vi "Automatic_light_attempt.vi"() -> ()   [LabVIEW 2019]
uses:
  <vilib>/MakerHub/LINX/Public/Peripherals/Analog/Analog Read 1 Chan.vi
  <vilib>/MakerHub/LINX/Public/Peripherals/Digital/Digital Write 1 Chan.vi
  <vilib>/MakerHub/LINX/Public/Peripherals/Analog/Analog Read N Chans.vi
  <vilib>/MakerHub/LINX/Public/Peripherals/Digital/Digital Write N Chans.vi
  <vilib>/MakerHub/LINX/Private/Local IO/LinxAnalogRead.vi
  <vilib>/MakerHub/LINX/Public/Utilities/Check Channel.vi
  <vilib>/MakerHub/LINX/Private/Local IO/LinxDigitalWrite.vi
  <vilib>/MakerHub/LINX/Public/Utilities/Open Serial.vi
  <vilib>/MakerHub/LINX/Private/Utilties/Generate Error.vi
  <vilib>/MakerHub/LINX/LMH-LINX.lvlib
panel:
  out "x < y?":bool
  out "Analog Output":dbl
  in  "stop":bool
  in  "Analog Channel":u8
  in  "Error In":errorcluster
  in  "Serial Port":refnum<visa-resource-name>="N/A"
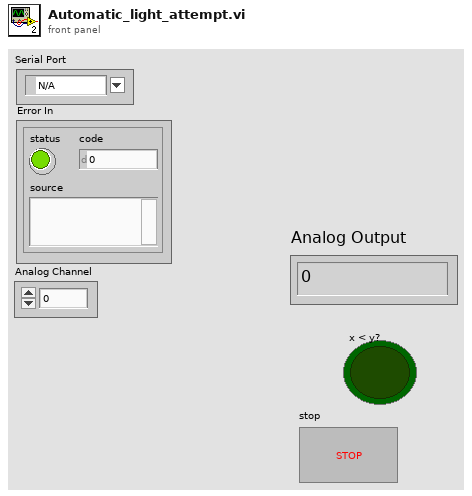
[diagram p1: front panel]
types:
  T1 = typedef "LMH-LINX.lvlib/LINX Ref.ctl" = cluster{"IO":T2, "Interface":T3, "LINX Device Config":T4}
  T2 = typedef "LMH-LINX.lvlib/Platform.ctl" = enum16{"Remote", "Local"}
  T3 = typedef "LMH-LINX.lvlib/Interface.ctl" = enum16{"Serial", "TCP"}
  T4 = typedef "LMH-LINX.lvlib/Device.lvlib/LINX Device Config.ctl" = cluster{"Interface":T3, "COM Port":refnum<visa-resource-name>, "TCP Configuration":T5, "Device Family":u8, "Device ID":u8, "Device Name":string, "TCP Ref":refnum<k5>, "Channels":T6}
  T5 = typedef "LMH-LINX.lvlib/Device.lvlib/TCP Config.ctl" = cluster{"IP Address":string, "Port":u16}
  T6 = typedef "LMH-LINX.lvlib/Channels.ctl" = cluster{"DI":u8[], "DO":u8[], "AI":u8[], "AO":u8[], "PWM":u8[], "QE":u8[], "UART":u8[], "I2C 2":u8[], "SPI":u8[], "CAN":u8[], "Servo":u8[], "AI Ref (V)":dbl, "AI Resolution (Bits)":u8, "AO Ref (V)":dbl, "AO Resolution (Bits)":u8}
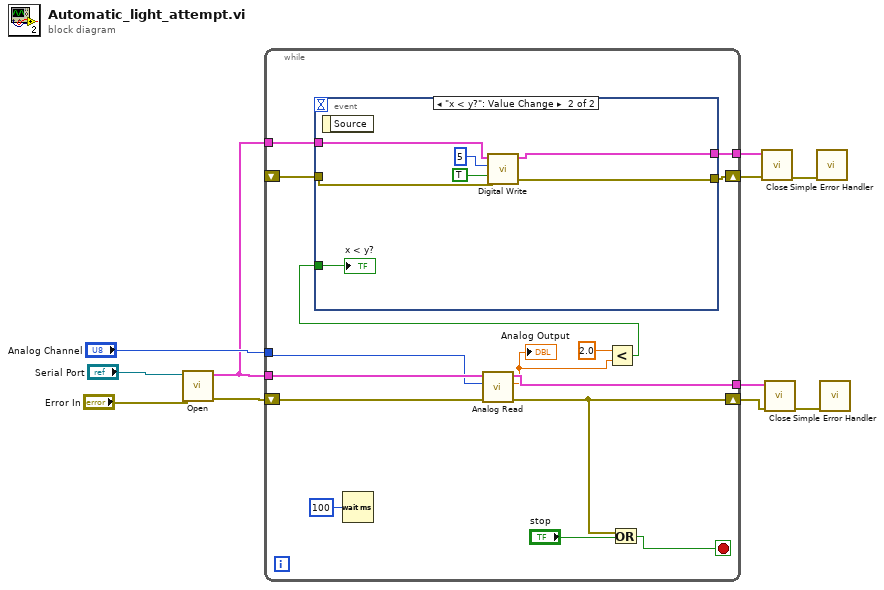
[diagram p0: block diagram]
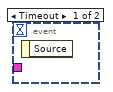
[diagram p2: hidden frame]
diagram:
  n1 = call-poly <vilib>:"Open.vi"("Error In"="Error In", "Serial Port"="Serial Port") -> ("Error Out"=w10:errorcluster, "LINX Resource"=w4:T1)  [unwired: 7 in, 1 out]
  n2 = while {
    tunnel: w4 -> [w26]
    tunnel: [w25] -> w11
    tunnel: "Analog Channel" -> [w23]
    shift-right: [w20] -> w9
    shift-left: w10 -> [w24]
    shift-right: [w15] -> w2
    shift-left: _ -> [w14]
    tunnel: w4 -> [w13]
    tunnel: [w12] -> w1
    stop <- w22 stop-if-true
    n3 = Wait (ms)(milliseconds to wait=u32 100) -> ()  [unwired: 1 out]
    n4 = call-poly <vilib>:"Analog Read.vi"("Error In"=w24, "Analog Channel"=w23, "LINX Resource"=w26) -> ("Error Out"=w20:errorcluster, "Voltage"=w18:dbl, "LINX Resource"=w25:T1)  [unwired: 5 in, 1 out]
    "Analog Output" <- w18
    n5 = Less?(x=2.0, y=w18) -> (x < y?=w16:bool)
    n6 = event shown="[1] \"x < y?\": Value Change" {
      selector: _ -> [_ _]
      dyn-events: _ -> [_ _]
      timeout: _ -> [_ _]
      tunnel: w16 -> [_ w33]
      tunnel: w14 -> [_ w32]
      tunnel: [_ w31] -> w15
      tunnel: w13 -> [_ w28]
      tunnel: [_ w27] -> w12
      event Timeout {
        n7 = event-data() -> ()  [unwired: 1 in, 1 out]
      }
      event "x < y?": Value Change {
        n8 = event-data() -> ()  [unwired: 1 in, 1 out]
        n9 = call-poly <vilib>:"Digital Write.vi"("Error In"=w32, "Output Value"=TRUE, "DO Channel"=u8 5, "LINX Resource"=w28) -> ("Error Out"=w31:errorcluster, "LINX Resource"=w27:T1)  [unwired: 6 in]
        "x < y?" <- w33
      }
    }
    n10 = Or(x=w20, y="stop") -> (x .or. y?=w22:bool)
  }
  n11 = call <vilib>:"Close.vi"("Error In"=w2, "LINX Resource"=w1) -> ("Error Out"=w3:errorcluster)  [unwired: 9 in]
  n12 = call <vilib>:"Close.vi"("Error In"=w9, "LINX Resource"=w11) -> ("Error Out"=w7:errorcluster)  [unwired: 9 in]
  n13 = call <vilib>:"Simple Error Handler.vi"("error in (no error)"=w3) -> ()  [unwired: 4 in, 5 out]
  n14 = call <vilib>:"Simple Error Handler.vi"("error in (no error)"=w7) -> ()  [unwired: 4 in, 5 out]
